vi "Drawer_2.vi"() -> ()   [LabVIEW 2014]
uses:
  <vilib>/Utility/file.llb/Read From Spreadsheet File (string).vi
  <vilib>/Utility/file.llb/Read From Spreadsheet File (I64).vi
  <vilib>/Utility/file.llb/Read From Spreadsheet File (DBL).vi
  <vilib>/Utility/file.llb/Write To Spreadsheet File (DBL).vi
  <vilib>/gmath/NI_Gmath.lvlib
panel:
  out "HF/LF_ERP 2":dbl[](graph)
  out "HF/LF slope":cluster{dbl[], dbl[]}[](graph)
  out "HF/LF flat":cluster{dbl[], dbl[]}[](graph)
  out "HF/LF_ERP":dbl[][](graph)
  out "HF_ERP":dbl[][](graph)
  out "LF_ERP":dbl[][](graph)
  out "VLF_ERP":dbl[][](graph)
  out "피험자_이름":string
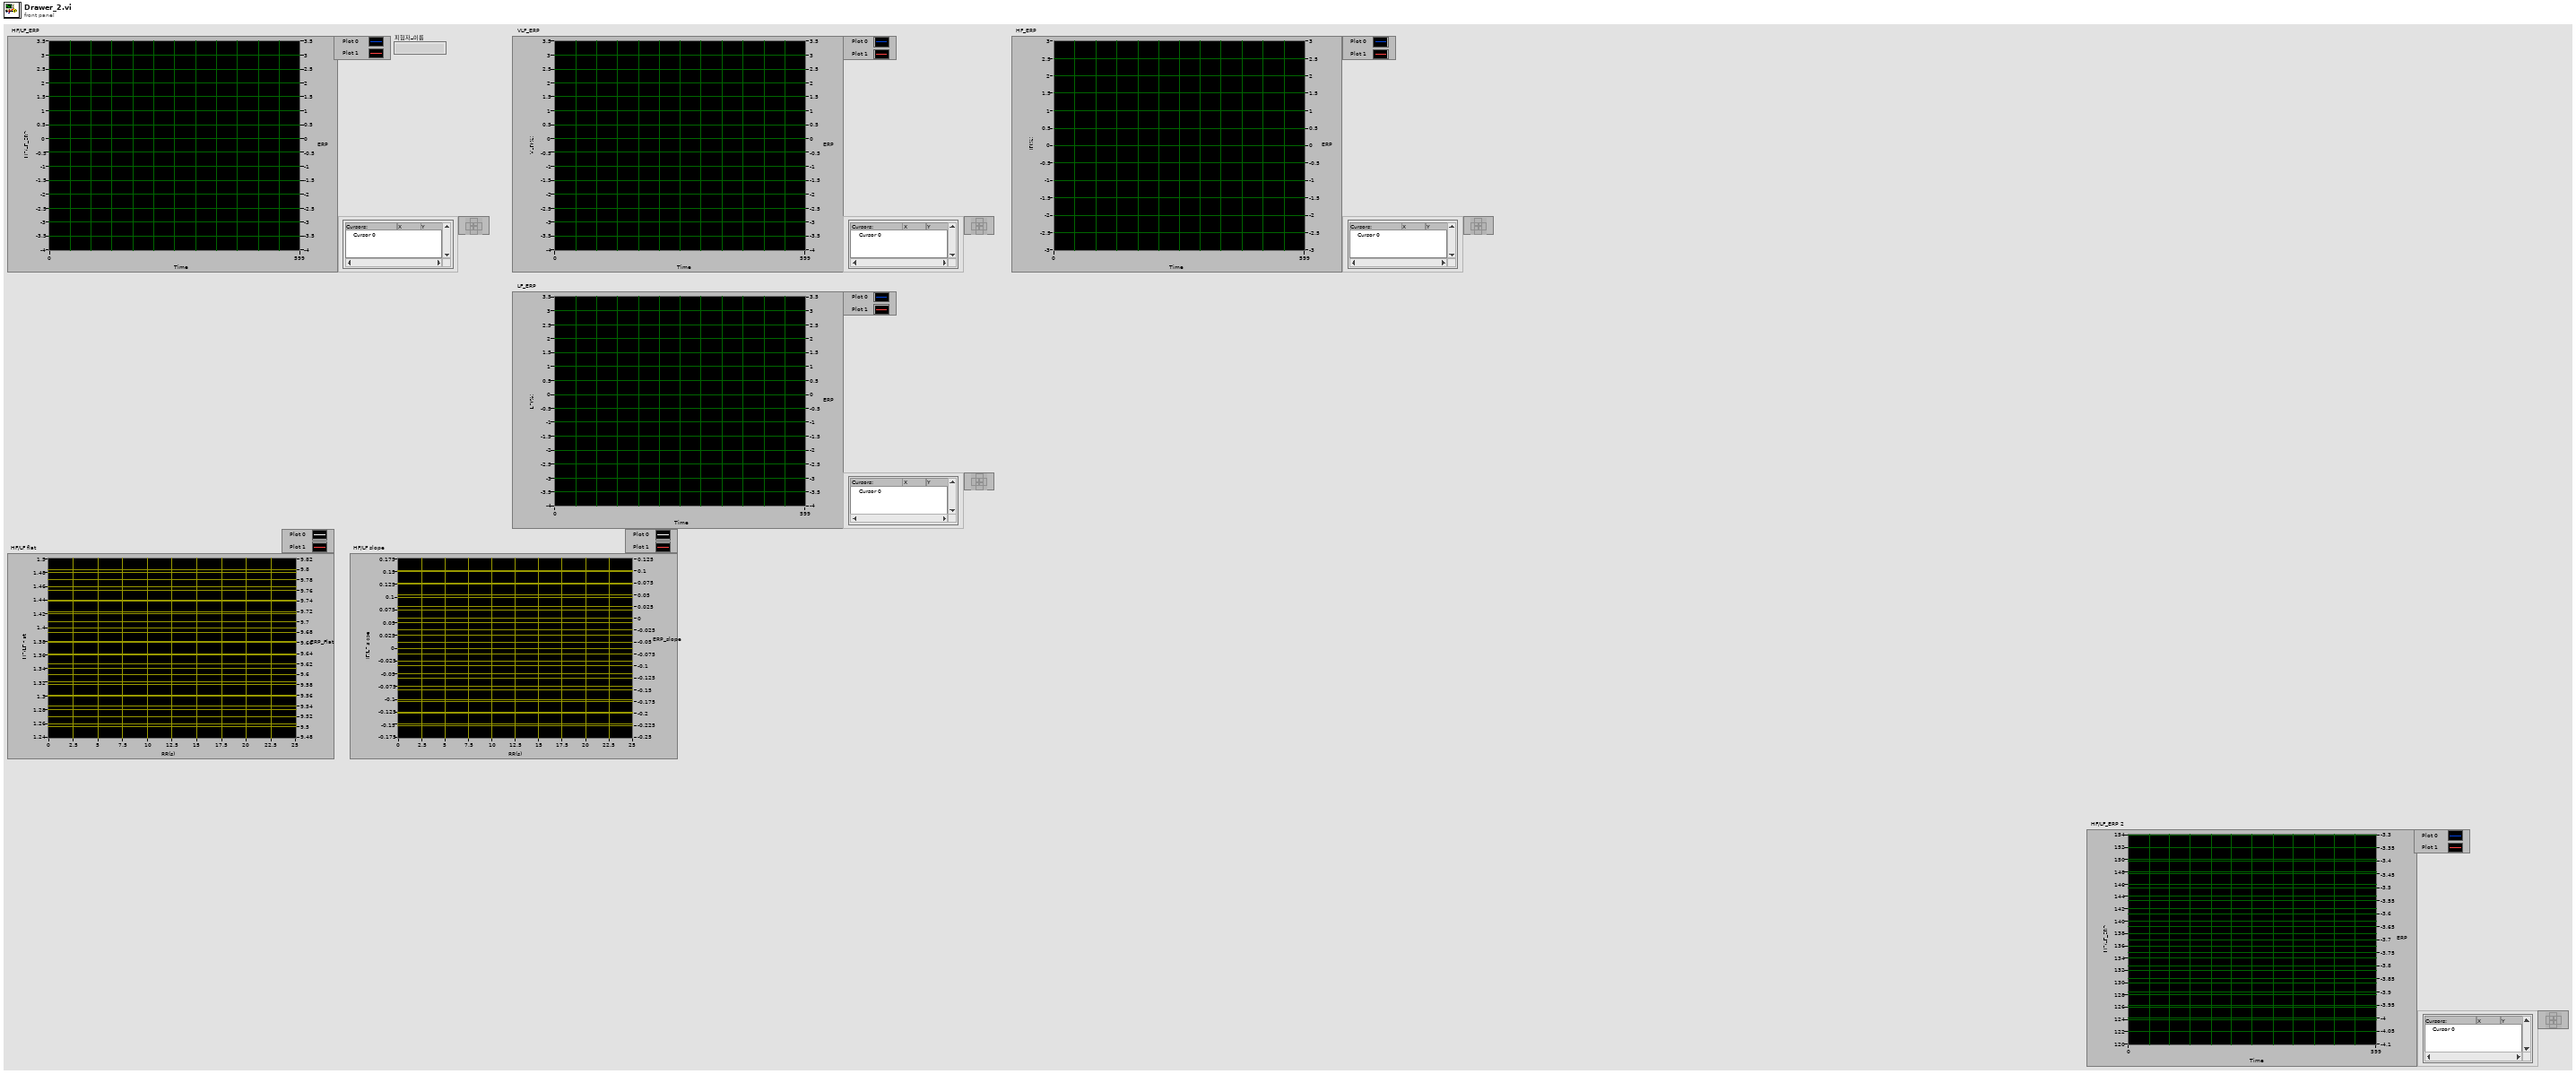
[diagram p1: front panel]
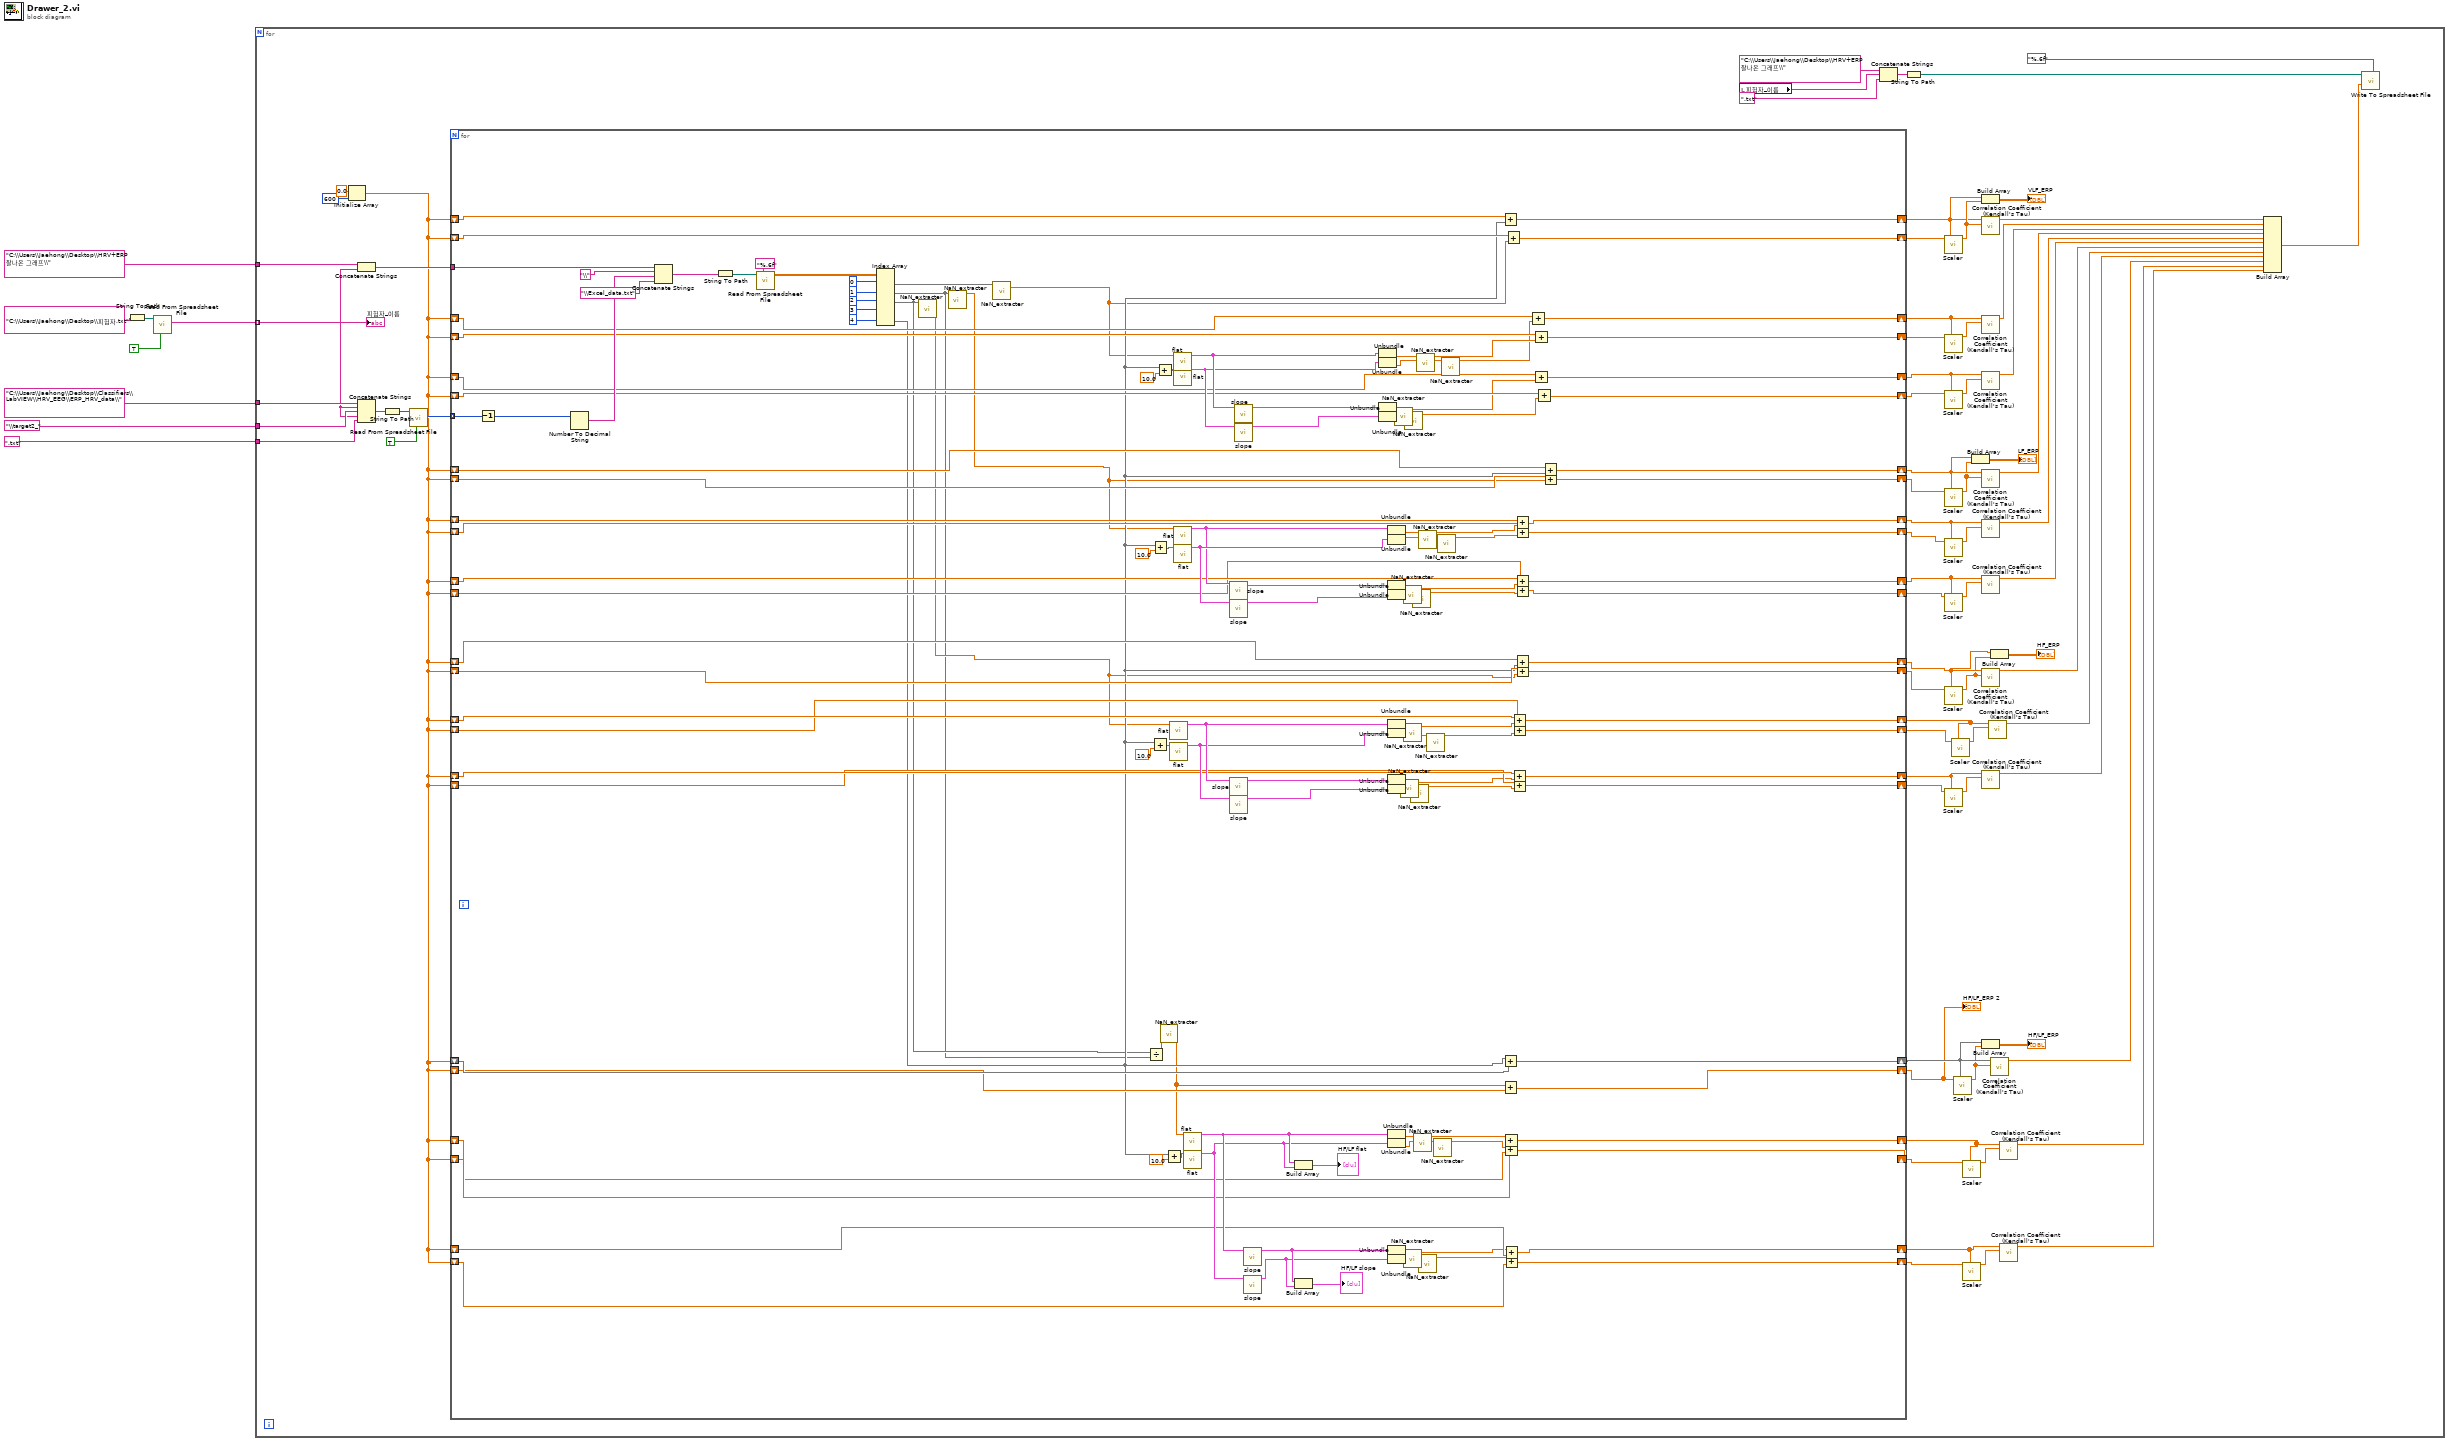
[diagram p0: block diagram]
diagram:
  n1 = String To Path(string="C:\\Users\\Jaehong\\Desktop\\피험자.txt") -> (path=w1:path)
  n2 = call-poly <vilib>:"Read From Spreadsheet File.vi"("transpose (no:F)"=TRUE, "file path (dialog if empty)"=w1) -> ("first row"=w3:string[])  [unwired: 5 in, 4 out]
  n3 = for {
    tunnel: "C:\\Users\\Jaehong\\Desktop\\HRV+ERP 잘나온 그래프\\" -> [w80]
    tunnel: "C:\\Users\\Jaehong\\Desktop\\Classifiers\\LabVIEW\\HRV_EEG\\ERP_HRV_data\\" -> [w78]
    tunnel: "\\target2_" -> [w77]
    tunnel: ".txt" -> [w76]
    tunnel: w3 -> [w74] mode=indexing
    n4 = Initialize Array(0.0 ("element"), 600 ("dimension size")) -> (w62:dbl[])
    n5 = Concatenate Strings(w80, w74) -> (w79:string)
    n6 = Concatenate Strings(w78, w74, w77, w74, w76) -> (w75:string)
    n7 = String To Path(string=w75) -> (path=w67:path)
    n8 = call-poly <vilib>:"Read From Spreadsheet File.vi"("transpose (no:F)"=TRUE, "file path (dialog if empty)"=w67) -> ("first row"=w65:i64[])  [unwired: 5 in, 4 out]
    n9 = for {
      tunnel: w79 -> [w210]
      tunnel: w65 -> [w177] mode=indexing
      shift-right: [w106] -> w21
      shift-left: w62 -> [w153]
      shift-right: [w104] -> w61
      shift-left: w62 -> [w152]
      shift-right: [w151] -> w58
      shift-left: w62 -> [w129]
      shift-right: [w150] -> w59
      shift-left: w62 -> [w128]
      shift-right: [w149] -> w55
      shift-left: w62 -> [w127]
      shift-right: [w148] -> w56
      shift-left: w62 -> [w126]
      shift-right: [w147] -> w25
      shift-left: w62 -> [w125]
      shift-right: [w130] -> w54
      shift-left: w62 -> [w124]
      shift-right: [w146] -> w52
      shift-left: w62 -> [w123]
      shift-right: [w145] -> w51
      shift-left: w62 -> [w122]
      shift-right: [w144] -> w49
      shift-left: w62 -> [w121]
      shift-right: [w143] -> w48
      shift-left: w62 -> [w120]
      shift-right: [w142] -> w31
      shift-left: w62 -> [w119]
      shift-right: [w141] -> w47
      shift-left: w62 -> [w118]
      shift-right: [w140] -> w45
      shift-left: w62 -> [w117]
      shift-right: [w139] -> w44
      shift-left: w62 -> [w116]
      shift-right: [w138] -> w42
      shift-left: w62 -> [w115]
      shift-right: [w137] -> w41
      shift-left: w62 -> [w114]
      shift-right: [w136] -> w28
      shift-left: w62 -> [w113]
      shift-right: [w135] -> w9
      shift-left: w62 -> [w112]
      shift-right: [w134] -> w11
      shift-left: w62 -> [w111]
      shift-right: [w133] -> w40
      shift-left: w62 -> [w110]
      shift-right: [w132] -> w38
      shift-left: w62 -> [w109]
      shift-right: [w131] -> w37
      shift-left: w62 -> [w108]
      n10 = Decrement(x=w177) -> (x-1=w107:i64)
      n11 = Number To Decimal String(number=w107) -> (decimal integer string=w208:string)  [unwired: 1 in]
      n12 = Concatenate Strings(w210, "\\", w208, "\\Excel_data.txt") -> (w206:string)
      n13 = String To Path(string=w206) -> (path=w205:path)
      n14 = call-poly <vilib>:"Read From Spreadsheet File.vi"("format (%.3f)"="%.6f", "file path (dialog if empty)"=w205) -> ("all rows"=w203:dbl[][])  [unwired: 5 in, 4 out]
      n15 = Index Array(array=w203, index (row) #1=0 ("index (row)"), index (row) #2=1 ("index (row)"), index (row) #3=2 ("index (row)"), index (row) #4=3 ("index (row)"), index (row) #5=4 ("index (row)")) -> (element #1=w103:dbl[], element #2=w82:dbl[], element #3=w84:dbl[], element #5=w105:dbl[])  [unwired: 5 in, 1 out]
      n16 = call "NaN_extracter.vi"("Array 1"=w84) -> ("Array 2"=w83:dbl[])  [unwired: 10 in]
      n17 = call "NaN_extracter.vi"("Array 1"=w82) -> ("Array 2"=w81:dbl[])  [unwired: 10 in]
      n18 = call "NaN_extracter.vi"("Array 1"=w103) -> ("Array 2"=w102:dbl[])  [unwired: 10 in]
      n19 = Divide(x=w84, y=w82) -> (x/y=w158:dbl[])
      n20 = Add(x=w105, y=10.0) -> (x+y=w195:dbl[])
      n21 = Add(x=w105, y=10.0) -> (x+y=w193:dbl[])
      n22 = Add(x=w105, y=10.0) -> (x+y=w191:dbl[])
      n23 = call "NaN_extracter.vi"("Array 1"=w158) -> ("Array 2"=w85:dbl[])  [unwired: 10 in]
      n24 = Add(x=w105, y=10.0) -> (x+y=w197:dbl[])
      n25 = call "flat.vi"("Input"=w83) -> ("XY Graph 3"=w181:cluster{dbl[], dbl[]})  [unwired: 10 in]
      n26 = call "flat.vi"("Input"=w195) -> ("XY Graph 3"=w180:cluster{dbl[], dbl[]})  [unwired: 10 in]
      n27 = call "flat.vi"("Input"=w102) -> ("XY Graph 3"=w189:cluster{dbl[], dbl[]})  [unwired: 10 in]
      n28 = call "flat.vi"("Input"=w191) -> ("XY Graph 3"=w188:cluster{dbl[], dbl[]})  [unwired: 10 in]
      n29 = call "flat.vi"("Input"=w81) -> ("XY Graph 3"=w184:cluster{dbl[], dbl[]})  [unwired: 10 in]
      n30 = call "flat.vi"("Input"=w193) -> ("XY Graph 3"=w185:cluster{dbl[], dbl[]})  [unwired: 10 in]
      n31 = call "flat.vi"("Input"=w85) -> ("XY Graph 3"=w176:cluster{dbl[], dbl[]})  [unwired: 10 in]
      n32 = call "flat.vi"("Input"=w197) -> ("XY Graph 3"=w175:cluster{dbl[], dbl[]})  [unwired: 10 in]
      n33 = call "slope.vi"("input"=w184) -> ("output"=w183:cluster{dbl[], dbl[]})  [unwired: 10 in]
      n34 = call "slope.vi"("input"=w185) -> ("output"=w182:cluster{dbl[], dbl[]})  [unwired: 10 in]
      n35 = call "slope.vi"("input"=w181) -> ("output"=w179:cluster{dbl[], dbl[]})  [unwired: 10 in]
      n36 = call "slope.vi"("input"=w180) -> ("output"=w178:cluster{dbl[], dbl[]})  [unwired: 10 in]
      n37 = call "slope.vi"("input"=w189) -> ("output"=w186:cluster{dbl[], dbl[]})  [unwired: 10 in]
      n38 = call "slope.vi"("input"=w188) -> ("output"=w187:cluster{dbl[], dbl[]})  [unwired: 10 in]
      n39 = call "slope.vi"("input"=w176) -> ("output"=w173:cluster{dbl[], dbl[]})  [unwired: 10 in]
      n40 = call "slope.vi"("input"=w175) -> ("output"=w172:cluster{dbl[], dbl[]})  [unwired: 10 in]
      n41 = Build Array(w176, w175) -> (→"HF/LF flat":cluster{dbl[], dbl[]}[])
      n42 = Build Array(w173, w172) -> (→"HF/LF slope":cluster{dbl[], dbl[]}[])
      n43 = Unbundle(w189) -> (w170:dbl[])  [unwired: 1 out]
      n44 = Unbundle(w188) -> (w169:dbl[])  [unwired: 1 out]
      n45 = Unbundle(w186) -> (w167:dbl[])  [unwired: 1 out]
      n46 = Unbundle(w187) -> (w168:dbl[])  [unwired: 1 out]
      n47 = Unbundle(w184) -> (w165:dbl[])  [unwired: 1 out]
      n48 = Unbundle(w185) -> (w166:dbl[])  [unwired: 1 out]
      n49 = Unbundle(w183) -> (w163:dbl[])  [unwired: 1 out]
      n50 = Unbundle(w182) -> (w164:dbl[])  [unwired: 1 out]
      n51 = Unbundle(w181) -> (w161:dbl[])  [unwired: 1 out]
      n52 = Unbundle(w180) -> (w162:dbl[])  [unwired: 1 out]
      n53 = Unbundle(w179) -> (w159:dbl[])  [unwired: 1 out]
      n54 = Unbundle(w178) -> (w160:dbl[])  [unwired: 1 out]
      n55 = Unbundle(w176) -> (w157:dbl[])  [unwired: 1 out]
      n56 = Unbundle(w175) -> (w156:dbl[])  [unwired: 1 out]
      n57 = Unbundle(w173) -> (w155:dbl[])  [unwired: 1 out]
      n58 = Unbundle(w172) -> (w154:dbl[])  [unwired: 1 out]
      n59 = call "NaN_extracter.vi"("Array 1"=w167) -> ("Array 2"=w99:dbl[])  [unwired: 10 in]
      n60 = call "NaN_extracter.vi"("Array 1"=w159) -> ("Array 2"=w91:dbl[])  [unwired: 10 in]
      n61 = call "NaN_extracter.vi"("Array 1"=w163) -> ("Array 2"=w95:dbl[])  [unwired: 10 in]
      n62 = call "NaN_extracter.vi"("Array 1"=w161) -> ("Array 2"=w93:dbl[])  [unwired: 10 in]
      n63 = call "NaN_extracter.vi"("Array 1"=w155) -> ("Array 2"=w87:dbl[])  [unwired: 10 in]
      n64 = call "NaN_extracter.vi"("Array 1"=w168) -> ("Array 2"=w98:dbl[])  [unwired: 10 in]
      n65 = call "NaN_extracter.vi"("Array 1"=w160) -> ("Array 2"=w90:dbl[])  [unwired: 10 in]
      n66 = call "NaN_extracter.vi"("Array 1"=w164) -> ("Array 2"=w94:dbl[])  [unwired: 10 in]
      n67 = call "NaN_extracter.vi"("Array 1"=w157) -> ("Array 2"=w89:dbl[])  [unwired: 10 in]
      n68 = call "NaN_extracter.vi"("Array 1"=w170) -> ("Array 2"=w101:dbl[])  [unwired: 10 in]
      n69 = call "NaN_extracter.vi"("Array 1"=w165) -> ("Array 2"=w97:dbl[])  [unwired: 10 in]
      n70 = call "NaN_extracter.vi"("Array 1"=w154) -> ("Array 2"=w86:dbl[])  [unwired: 10 in]
      n71 = call "NaN_extracter.vi"("Array 1"=w162) -> ("Array 2"=w92:dbl[])  [unwired: 10 in]
      n72 = call "NaN_extracter.vi"("Array 1"=w156) -> ("Array 2"=w88:dbl[])  [unwired: 10 in]
      n73 = call "NaN_extracter.vi"("Array 1"=w166) -> ("Array 2"=w96:dbl[])  [unwired: 10 in]
      n74 = call "NaN_extracter.vi"("Array 1"=w169) -> ("Array 2"=w100:dbl[])  [unwired: 10 in]
      n75 = Add(x=w153, y=w105) -> (x+y=w106:dbl[])
      n76 = Add(x=w105, y=w113) -> (x+y=w136:dbl[])
      n77 = Add(x=w85, y=w112) -> (x+y=w135:dbl[])
      n78 = Add(x=w89, y=w111) -> (x+y=w134:dbl[])
      n79 = Add(x=w88, y=w110) -> (x+y=w133:dbl[])
      n80 = Add(x=w87, y=w109) -> (x+y=w132:dbl[])
      n81 = Add(x=w86, y=w108) -> (x+y=w131:dbl[])
      n82 = Add(x=w152, y=w102) -> (x+y=w104:dbl[])
      n83 = Add(x=w117, y=w93) -> (x+y=w140:dbl[])
      n84 = Add(x=w116, y=w92) -> (x+y=w139:dbl[])
      n85 = Add(x=w115, y=w91) -> (x+y=w138:dbl[])
      n86 = Add(x=w114, y=w90) -> (x+y=w137:dbl[])
      n87 = Add(x=w123, y=w97) -> (x+y=w146:dbl[])
      n88 = Add(x=w122, y=w96) -> (x+y=w145:dbl[])
      n89 = Add(x=w121, y=w95) -> (x+y=w144:dbl[])
      n90 = Add(x=w120, y=w94) -> (x+y=w143:dbl[])
      n91 = Add(x=w119, y=w105) -> (x+y=w142:dbl[])
      n92 = Add(x=w118, y=w83) -> (x+y=w141:dbl[])
      n93 = Add(x=w129, y=w100) -> (x+y=w151:dbl[])
      n94 = Add(x=w128, y=w101) -> (x+y=w150:dbl[])
      n95 = Add(x=w127, y=w99) -> (x+y=w149:dbl[])
      n96 = Add(x=w126, y=w98) -> (x+y=w148:dbl[])
      n97 = Add(x=w125, y=w105) -> (x+y=w147:dbl[])
      n98 = Add(x=w124, y=w81) -> (x+y=w130:dbl[])
    }
    "HF/LF_ERP 2" <- w9
    n99 = local read "피험자_이름"() -> (w72:string)
    n100 = Concatenate Strings("C:\\Users\\Jaehong\\Desktop\\HRV+ERP 잘나온 그래프\\", w72, ".txt") -> (w70:string)
    n101 = String To Path(string=w70) -> (path=w69:path)
    n102 = call "Scaler.vi"("Array1"=w21, "Array2"=w61) -> ("Array_out"=w22:dbl[])  [unwired: 9 in]
    n103 = call "Scaler.vi"("Array1"=w58, "Array2"=w59) -> ("Array_out"=w60:dbl[])  [unwired: 9 in]
    n104 = call "Scaler.vi"("Array1"=w55, "Array2"=w56) -> ("Array_out"=w57:dbl[])  [unwired: 9 in]
    n105 = call "Scaler.vi"("Array1"=w25, "Array2"=w54) -> ("Array_out"=w24:dbl[])  [unwired: 9 in]
    n106 = call "Scaler.vi"("Array1"=w52, "Array2"=w51) -> ("Array_out"=w53:dbl[])  [unwired: 9 in]
    n107 = call "Scaler.vi"("Array1"=w49, "Array2"=w48) -> ("Array_out"=w50:dbl[])  [unwired: 9 in]
    n108 = call "Scaler.vi"("Array1"=w31, "Array2"=w47) -> ("Array_out"=w30:dbl[])  [unwired: 9 in]
    n109 = call "Scaler.vi"("Array1"=w42, "Array2"=w41) -> ("Array_out"=w43:dbl[])  [unwired: 9 in]
    n110 = call "Scaler.vi"("Array1"=w45, "Array2"=w44) -> ("Array_out"=w46:dbl[])  [unwired: 9 in]
    n111 = call "Scaler.vi"("Array1"=w28, "Array2"=w9) -> ("Array_out"=w27:dbl[])  [unwired: 9 in]
    n112 = call "Scaler.vi"("Array1"=w11, "Array2"=w40) -> ("Array_out"=w10:dbl[])  [unwired: 9 in]
    n113 = call "Scaler.vi"("Array1"=w38, "Array2"=w37) -> ("Array_out"=w39:dbl[])  [unwired: 9 in]
    n114 = Build Array(w25, w24) -> (→"LF_ERP":dbl[][])
    n115 = Build Array(w21, w22) -> (→"VLF_ERP":dbl[][])
    n116 = call <vilib>:"Correlation Coefficient (Kendall's Tau).vi"("Y"=w22, "X"=w21) -> ("correlation coefficient r"=w36:dbl)  [unwired: 8 in, 1 out]
    n117 = call <vilib>:"Correlation Coefficient (Kendall's Tau).vi"("Y"=w60, "X"=w58) -> ("correlation coefficient r"=w35:dbl)  [unwired: 8 in, 1 out]
    n118 = call <vilib>:"Correlation Coefficient (Kendall's Tau).vi"("Y"=w57, "X"=w55) -> ("correlation coefficient r"=w34:dbl)  [unwired: 8 in, 1 out]
    n119 = call <vilib>:"Correlation Coefficient (Kendall's Tau).vi"("Y"=w24, "X"=w25) -> ("correlation coefficient r"=w20:dbl)  [unwired: 8 in, 1 out]
    n120 = call <vilib>:"Correlation Coefficient (Kendall's Tau).vi"("Y"=w53, "X"=w52) -> ("correlation coefficient r"=w19:dbl)  [unwired: 8 in, 1 out]
    n121 = call <vilib>:"Correlation Coefficient (Kendall's Tau).vi"("Y"=w50, "X"=w49) -> ("correlation coefficient r"=w18:dbl)  [unwired: 8 in, 1 out]
    n122 = call <vilib>:"Correlation Coefficient (Kendall's Tau).vi"("Y"=w30, "X"=w31) -> ("correlation coefficient r"=w17:dbl)  [unwired: 8 in, 1 out]
    n123 = call <vilib>:"Correlation Coefficient (Kendall's Tau).vi"("Y"=w43, "X"=w42) -> ("correlation coefficient r"=w15:dbl)  [unwired: 8 in, 1 out]
    n124 = Build Array(w28, w27) -> (→"HF/LF_ERP":dbl[][])
    n125 = call <vilib>:"Correlation Coefficient (Kendall's Tau).vi"("Y"=w46, "X"=w45) -> ("correlation coefficient r"=w16:dbl)  [unwired: 8 in, 1 out]
    n126 = Build Array(w31, w30) -> (→"HF_ERP":dbl[][])
    n127 = call <vilib>:"Correlation Coefficient (Kendall's Tau).vi"("Y"=w27, "X"=w28) -> ("correlation coefficient r"=w14:dbl)  [unwired: 8 in, 1 out]
    n128 = call <vilib>:"Correlation Coefficient (Kendall's Tau).vi"("Y"=w10, "X"=w11) -> ("correlation coefficient r"=w13:dbl)  [unwired: 8 in, 1 out]
    n129 = call <vilib>:"Correlation Coefficient (Kendall's Tau).vi"("Y"=w39, "X"=w38) -> ("correlation coefficient r"=w12:dbl)  [unwired: 8 in, 1 out]
    n130 = Build Array(w36, w35, w34, w20, w19, w18, w17, w16, w15, w14, w13, w12) -> (w33:dbl[])
    n131 = call-poly <vilib>:"Write To Spreadsheet File.vi"("format (%.3f)"="%.6f", "1D data"=w33, "file path (dialog if empty)"=w69) -> ()  [unwired: 5 in, 1 out]
    "피험자_이름" <- w74
  }
